vi "estimador velocidade bola.vi"(11 "Detection Ball":T1) -> (2 "v_y (cm/s)":dbl, 3 "v_x (cm/s)":dbl)   [LabVIEW 2016]
uses:
  SSL Detection Ball.ctl
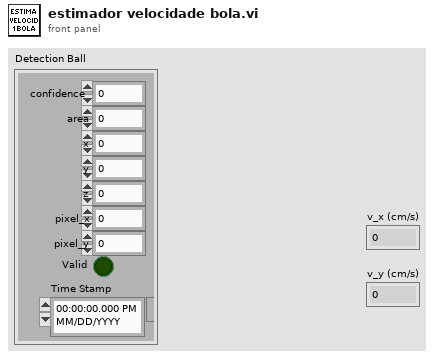
[diagram p1: front panel]
types:
  T1 = typedef "SSL Detection Ball.ctl" = cluster{"x":sgl, "area":u32, "confidence":sgl, "y":sgl, "z":sgl, "pixel_x":sgl, "pixel_y":sgl, "Valid":bool, "Time Stamp":timestamp}
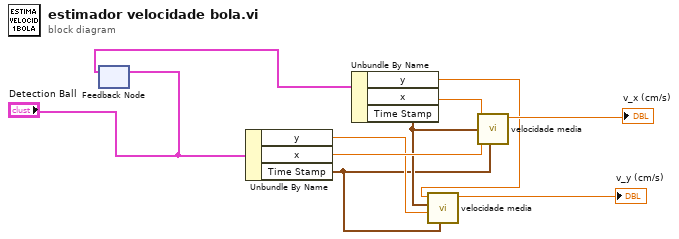
[diagram p0: block diagram]
diagram:
  n1 = feedback #1() -> (w10:T1)  [unwired: 1 in]
  n2 = feedback-in #1("Detection Ball") -> ()
  n3 = Unbundle By Name("Detection Ball") -> ("y"=w5:sgl, "x"=w8:sgl, "Time Stamp"=w2:timestamp)
  n4 = Unbundle By Name(w10) -> ("y"=w6:sgl, "x"=w9:sgl, "Time Stamp"=w3:timestamp)
  n5 = call "velocidade media.vi"("Time Stamp 2"=w2, "x 2"=w5, "Time Stamp 1"=w3, "x1"=w6) -> ("speed (cm/s)"=→"v_y (cm/s)":dbl)  [unwired: 7 in]
  n6 = call "velocidade media.vi"("Time Stamp 2"=w2, "x 2"=w8, "Time Stamp 1"=w3, "x1"=w9) -> ("speed (cm/s)"=→"v_x (cm/s)":dbl)  [unwired: 7 in]
